vi "Configure Acquisition Record.vi"(0 "VISA Resource Name":refnum<visa-resource-name>, 5 "Time Per Record (4.0e-3 s)":dbl=0.004 format="%.2p", 7 "Record Length (10000)":i32=10000, 9 "Acquisition Start Time (0.0 s)":dbl format="%.2p", 11 "error in (no error)":errorcluster {"code" format="%.0x"}) -> (4 "VISA Resource Name Out":refnum<visa-resource-name>, 15 "error out":errorcluster {"code" format="%.0x"})   [LabVIEW 2010, in "Tektronix TDS 3000 Series.lvlib"]
doc: "This VI configures the common properties of the acquisition subsystem. These properties are the time per record, record length, and acquisition start time."
uses:
  <instrlib>/Tektronix TDS 3000 Series/Tektronix TDS 3000 Series.lvlib
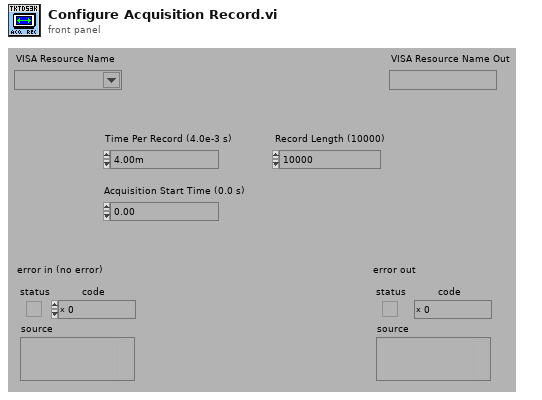
[diagram p1: front panel]
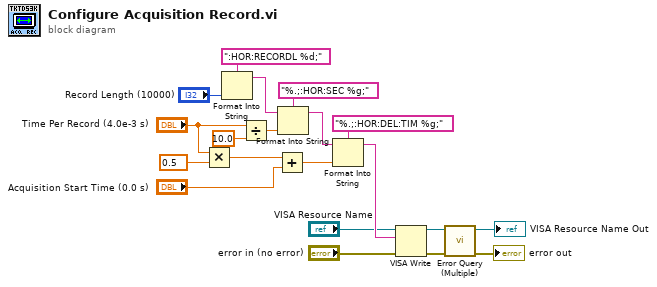
[diagram p0: block diagram]
diagram:
  n1 = Multiply(x="Time Per Record (4.0e-3 s)", y=0.5) -> (x*y=w12:dbl)
  n2 = Format Into String(format string=":HOR:RECORDL %d;", "Record Length (10000)") -> (resulting string=w5:string)  [unwired: 2 in, 1 out]
  n3 = Divide(x="Time Per Record (4.0e-3 s)", y=10.0) -> (x/y=w16:dbl)
  n4 = Add(x=w12, y="Acquisition Start Time (0.0 s)") -> (x+y=w14:dbl)
  n5 = Format Into String(format string="%.;:HOR:SEC %g;", initial string=w5, w16) -> (resulting string=w18:string)  [unwired: 1 in, 1 out]
  n6 = Format Into String(format string="%.;:HOR:DEL:TIM %g;", initial string=w18, w14) -> (resulting string=w17:string)  [unwired: 1 in, 1 out]
  n7 = VISA Write(VISA resource name="VISA Resource Name", write buffer=w17, error in (no error)="error in (no error)") -> (VISA resource name out=w4:refnum<visa-resource-name>, error out=w3:errorcluster)  [unwired: 1 out]
  n8 = call <instrlib>:"Error Query (Multiple).vi"("error in (no error)"=w3, "VISA Resource Name"=w4) -> ("error out"=→"error out":errorcluster, "VISA Resource Name Out"=→"VISA Resource Name Out":refnum<visa-resource-name>)  [unwired: 6 in, 2 out]
